vi "Get Events.vi"(11 "Create Project View in":refnum<class "Create Project View.lvclass">) -> (2 "Events":T1, 3 "Create Project View out":refnum<class "Create Project View.lvclass">)   [LabVIEW 2013, in "Create Project View.lvlib" / "Create Project View.lvclass"]
uses:
  Create Project View.lvclass
  Typedef/Events.ctl
  Create Project View.lvclass/Create Project View.ctl
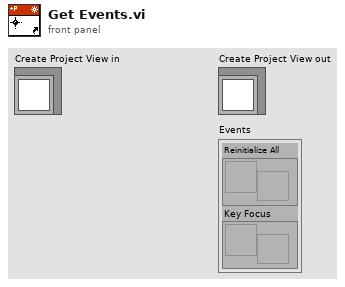
[diagram p1: front panel]
types:
  T1 = typedef "Create Project View.lvlib/Create Project View.lvclass/Events.ctl" = cluster{"Reinitialize All":refnum<user-event>, "Key Focus":refnum<user-event>}
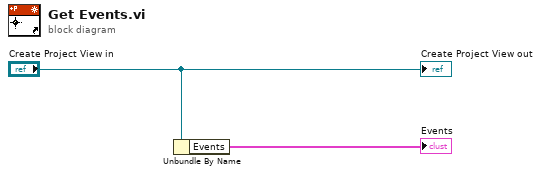
[diagram p0: block diagram]
diagram:
  n1 = Unbundle By Name("Create Project View in") -> ("Events"=→"Events":T1)
  "Create Project View out" <- "Create Project View in"
